vi "LRS Sums (FPGA w Pipelining).vi"(9 "max":i32, 10 "i":i32, 11 "DataIn":i16) -> (3 "DataOut":T1)   [LabVIEW 2015]
uses:
  <vilib>/Platform/TimedLoop/XDataNode/timing_clust.ctl
  <vilib>/Platform/TimedLoop/XDataNode/nitl_modes.ctl
  <vilib>/Platform/TimedLoop/XDataNode/wakeup.ctl
  <vilib>/rvi/Emulation/niFpgaGetClockAttributes.vi
  <vilib>/rvi/Emulation/niFpgaSctlEmulationGetInTimedLoop.vi
  <vilib>/rvi/Emulation/niFpgaEmulationReportErrorSimple.vi
  <vilib>/rvi/Emulation/niFpgaCriticalErrorInLSC.vi
  <vilib>/Platform/TimedLoop/XDataNode/XDataNode.xnode
  <vilib>/rvi/FXPMathLib/FxpAdd/XNode/nifxpmath_Add.xnode
  <vilib>/rvi/FXPMathLib/FxpMul/XNode/nifxpmath_Multiplier.xnode
  <vilib>/rvi/FXPMathLib/sim/FxpSim.dll
  <vilib>/Platform/TimedLoop/XDataNode/XDNodeRunTimeDep.lvlib
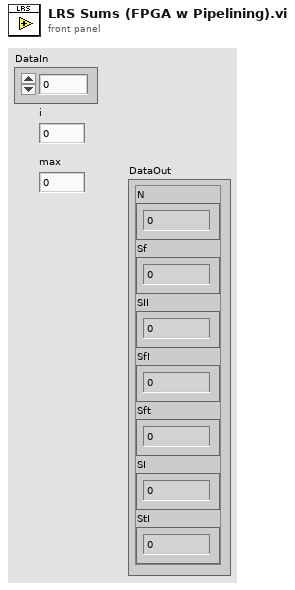
[diagram p1: front panel]
types:
  T1 = cluster{"fixed-point type":fxp<+/-,64,64>, "x+y":fxp<+/-,64,64>, "x+y":fxp<+/-,64,64>, "x+y":fxp<+/-,64,64>, "x+y":fxp<+/-,64,64>, "x+y":fxp<+/-,64,64>, "x+y":fxp<+/-,64,64>}
  T2 = typedef "XDNodeRunTimeDep.lvlib/timing_clust.ctl" = cluster{"Expected End [f-1]":u64, "Actual End [f-1]":u64, "Finished Late? [f-1]":bool, "Expected End [i-1]":u64, "Actual End [i-1]":u64, "Finished Late? [i-1]":bool, "Expected Start [i]":u64, "Actual Start [i]":u64, "Expected Start [f]":u64, "Actual Start [f]":u64, "Source Name":string, "Structure Name":string, "Period":i64, "Deadline":i64, "Offset":i64, "Start":i64, "Priority":i32, "Timeout":i32, "Mode":T3, "Wakeup Reason":T4, "Error":errorcluster, "Source Type":string, "Secondary Source Type":string, "Global End Time":u64, "Global Start Time":u64, "Frame Duration":u64, "Iteration Duration":u64, "Assigned CPU":i32, "I/O Scan Engine Mode":u32}
  T3 = typedef "XDNodeRunTimeDep.lvlib/nitl_modes.ctl" = enum32{"No Change", "Process missed periods, maintain original phase", "Discard missed periods, maintain original phase", "Process missed periods, ignore original phase", "Discard missed periods, ignore original phase"}
  T4 = typedef "XDNodeRunTimeDep.lvlib/wakeup.ctl" = enum32{"Normal", "Aborted", "Asynchronous wakeup", "Timing source error", "Timed loop error", "Timeout"}
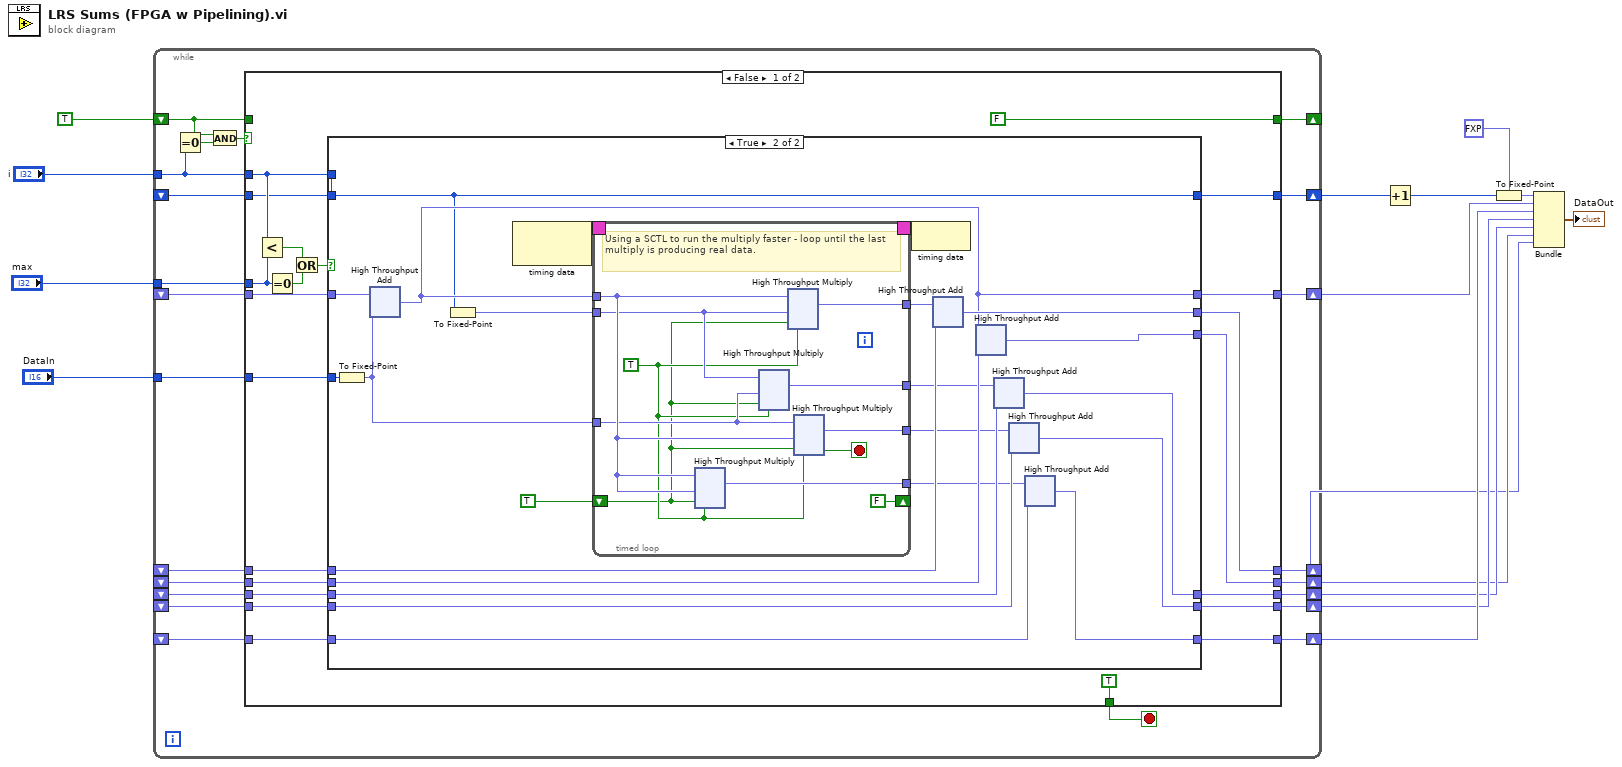
[diagram p0: block diagram]
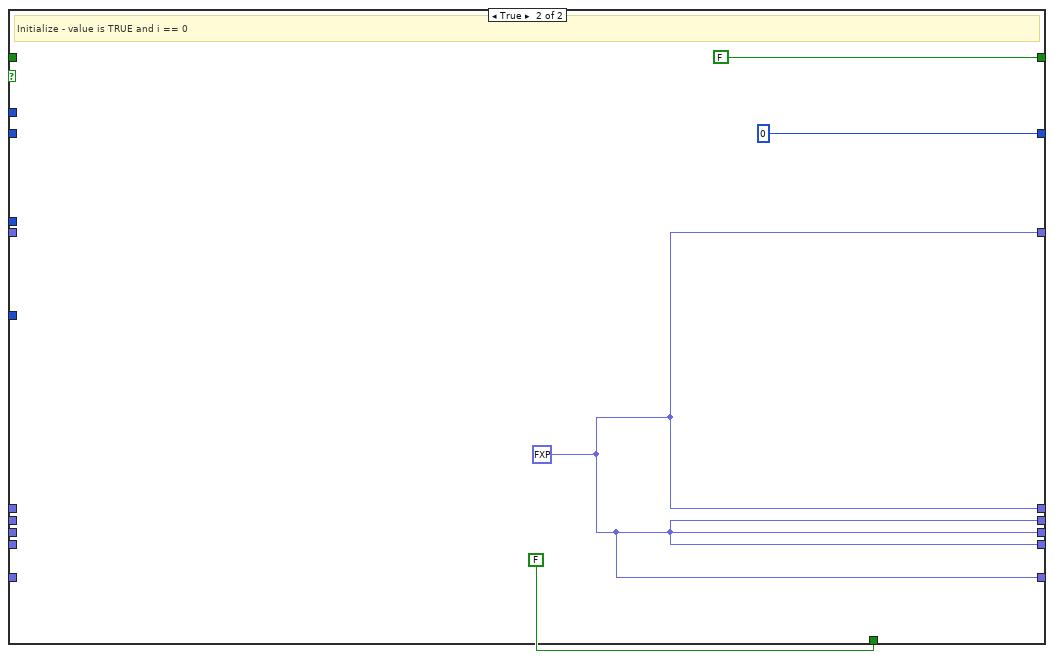
[diagram p3: hidden frame]
diagram:
  n1 = while {
    shift-right: [w37] -> w14
    shift-left: _ -> [w36]
    shift-right: [w35] -> w13
    shift-left: _ -> [w34]
    shift-right: [w23] -> w12
    shift-left: _ -> [w33]
    shift-right: [w32] -> w11
    shift-left: _ -> [w31]
    shift-right: [w30] -> w10
    shift-left: _ -> [w29]
    shift-right: [w28] -> w15
    shift-left: _ -> [w27]
    tunnel: "i" -> [w20]
    shift-right: [w25] -> w2
    shift-left: _ -> [w26]
    tunnel: "max" -> [w24]
    tunnel: "DataIn" -> [w22]
    shift-right: [w19] -> _
    shift-left: TRUE -> [w17]
    stop <- w21 stop-if-true
    n2 = Equal To 0?(x=w20) -> (x = 0?=w18:bool)
    n3 = And(x=w17, y=w18) -> (x .and. y?=w16:bool)
    n4 = case shown="False" w16 {
      tunnel: [w59 w105] -> w37
      tunnel: w36 -> [w58 _]
      tunnel: [w57 w105] -> w35
      tunnel: w34 -> [w56 _]
      tunnel: w33 -> [w55 _]
      tunnel: [w54 w105] -> w32
      tunnel: w31 -> [w53 _]
      tunnel: [w52 w105] -> w30
      tunnel: w29 -> [w51 _]
      tunnel: [w50 w105] -> w28
      tunnel: w27 -> [w49 _]
      tunnel: w20 -> [w46 _]
      tunnel: w26 -> [w44 _]
      tunnel: [w43 0] -> w25
      tunnel: w24 -> [w42 _]
      tunnel: [w41 w105] -> w23
      tunnel: w22 -> [w40 _]
      tunnel: [TRUE FALSE] -> w21
      tunnel: [FALSE FALSE] -> w19
      tunnel: w17 -> [_ _]
      frame False {
        n5 = Less?(x=w46, y=w42) -> (x < y?=w48:bool)
        n6 = Equal To 0?(x=w42) -> (x = 0?=w47:bool)
        n7 = Or(x=w48, y=w47) -> (x .or. y?=w45:bool)
        n8 = case shown="True" w45 {
          tunnel: [w60 w89] -> w59
          tunnel: w58 -> [w60 w88]
          tunnel: [w61 w87] -> w57
          tunnel: w56 -> [w61 w86]
          tunnel: [w62 w85] -> w41
          tunnel: w55 -> [w62 w84]
          tunnel: [w63 w83] -> w54
          tunnel: w53 -> [w63 w82]
          tunnel: [w64 w81] -> w52
          tunnel: w51 -> [w64 w80]
          tunnel: [w65 w79] -> w50
          tunnel: w49 -> [w65 w78]
          tunnel: w46 -> [_ w70]
          tunnel: w44 -> [w66 _]
          tunnel: [w66 w70] -> w43
          tunnel: w40 -> [_ w77]
          frame False {
            # "If max iterations is exceeded..."
          }
          frame True {
            n9 = To Fixed-Point(number=w77) -> (fixed-point=w76:fxp<+/-,16,16>)  [unwired: 1 in]
            n10 = xnode ("High Throughput Add")("x"=w78, "y"=w76) -> ("x+y"=w79:fxp<+/-,64,64>)
            n11 = To Fixed-Point(number=w70) -> (fixed-point=w75:fxp<+/-,32,32>)  [unwired: 1 in]
            n12 = node-c288() -> (w69:T2)  [unwired: 1 in]
            n13 = timed-loop {
              timing: w69 -> [_]
              timing-out: [_] -> w68
              tunnel: w79 -> [w100]
              tunnel: w76 -> [w99]
              tunnel: w75 -> [w98]
              tunnel: [w97] -> w74
              tunnel: [w96] -> w73
              tunnel: [w95] -> w72
              tunnel: [w94] -> w71
              shift-right: [FALSE] -> _
              shift-left: TRUE -> [w90]
              stop <- w92 stop-if-true
              w93 = TRUE ("ready for output (T)")
              # "Using a SCTL to run the multiply faster - loop until the last multiply is producing real data."
              n14 = xnode ("High Throughput Multiply")("x"=w100, "y"=w100, "input valid"=w90, "ready for output (T)"=w93) -> ("x*y"=w95:fxp<+/-,64,64>)  [unwired: 2 out]
              n15 = xnode ("High Throughput Multiply")("x"=w98, "y"=w99, "input valid"=w90, "ready for output (T)"=w93) -> ("x*y"=w97:fxp<+/-,64,64>)  [unwired: 2 out]
              n16 = xnode ("High Throughput Multiply")("x"=w100, "y"=w98, "input valid"=w90, "ready for output (T)"=w93) -> ("x*y"=w94:fxp<+/-,64,64>)  [unwired: 2 out]
              n17 = xnode ("High Throughput Multiply")("x"=w99, "y"=w100, "input valid"=w90, "ready for output (T)"=w93) -> ("x*y"=w96:fxp<+/-,64,64>, "output valid"=w92:bool)  [unwired: 1 out]
            }
            n18 = node-c288(w68) -> ()
            n19 = xnode ("High Throughput Add")("x"=w71, "y"=w80) -> ("x+y"=w81:fxp<+/-,64,64>)
            n20 = xnode ("High Throughput Add")("x"=w79, "y"=w82) -> ("x+y"=w83:fxp<+/-,64,64>)
            n21 = xnode ("High Throughput Add")("x"=w74, "y"=w84) -> ("x+y"=w85:fxp<+/-,64,64>)
            n22 = xnode ("High Throughput Add")("x"=w73, "y"=w86) -> ("x+y"=w87:fxp<+/-,64,64>)
            n23 = xnode ("High Throughput Add")("x"=w72, "y"=w88) -> ("x+y"=w89:fxp<+/-,64,64>)
          }
        }
      }
      frame True {
        w105 = fxp<+/-,48,48> 0.0 ("fixed-point type")
        # "Initialize - value is TRUE and i == 0"
      }
    }
  }
  n24 = Increment(x=w2) -> (x+1=w1:i32)
  n25 = To Fixed-Point(fixed-point type=fxp<+/-,64,64> 0.0, number=w1) -> (fixed-point=w5:fxp<+/-,64,64>)
  n26 = Bundle("fixed-point type"=w5, "x+y"=w15, "x+y"=w14, "x+y"=w13, "x+y"=w12, "x+y"=w11, "x+y"=w10) -> (→"DataOut":T1)  [unwired: 1 in]
